vi "ex2_2.vi"() -> ()   [LabVIEW 2017]
uses:
  <vilib>/Waveform/WDTOps.llb/WDT Append Waveforms DBL.vi
panel:
  out "Waveform Chart":waveform(dbl)(graph)
  in  "stop":bool
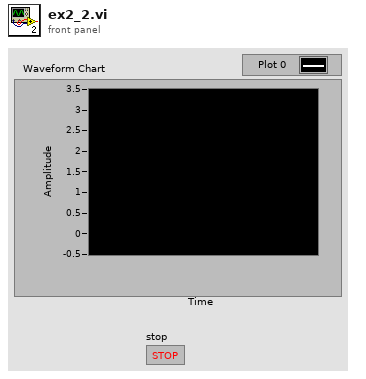
[diagram p1: front panel]
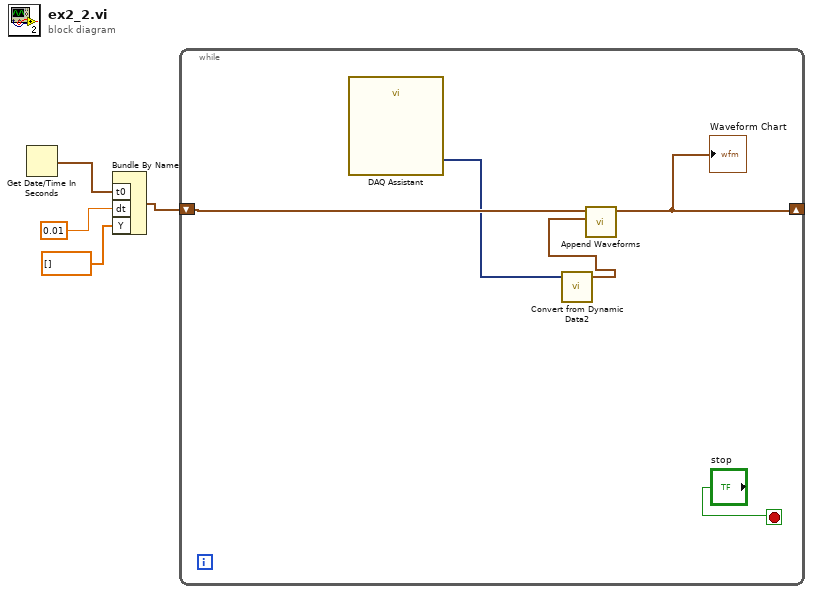
[diagram p0: block diagram]
diagram:
  n1 = Get Date/Time In Seconds() -> (seconds since 1Jan1904=w1:timestamp)
  n2 = Bundle By Name("t0"=w1, "dt"=0.01, "Y"=dbl[] []) -> (w4:waveform(dbl))  [unwired: 1 in]
  n3 = while {
    shift-right: [w8] -> _
    shift-left: w4 -> [w7]
    stop <- "stop" stop-if-true
    n4 = call "DAQ Assistant"() -> ("data"=w5:dynamicdata)  [unwired: 16 in, 3 out]
    n5 = call "Convert from Dynamic Data2"("Dynamic Data Type"=w5) -> ("Waveform"=w6:waveform(dbl))  [unwired: 3 in]
    n6 = call-poly <vilib>:"Append Waveforms.vi"("waveform B"=w6, "waveform A"=w7) -> ("waveform out"=w8:waveform(dbl))  [unwired: 8 in, 1 out]
    "Waveform Chart" <- w8
  }
